vi "Telemetry.vi"   [LabVIEW 2016]
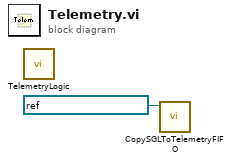
[diagram p0: block diagram]
diagram:
  n1 = call "TelemetryLogic.vi"() -> ()  [unwired: 12 in]
  n2 = call "CopySGLToTelemetryFIFO.vi"("SourceFIFO"=refnum<k21> "TelemetrySGLFIFO") -> ()  [unwired: 11 in]
